vi "Send Menu Selection.vi"(4 "Item Path":string, 5 "EventFilter Reference":T1, 6 "Item Tag":string, 7 "App Item?":bool, 8 "Time":u32, 9 "MenuRef":refnum<k9>, 10 "VI Refnum":refnum<vi>, 11 "Message Enqueuer in":refnum<class "Message Enqueuer.lvclass">) -> (0 "error out":errorcluster, 3 "Filtered EventDataMessage":refnum<class "MenuSelectionMsg.lvclass">)   [LabVIEW 2018, in "MVA Framework.lvlib" / "ActorEvents.lvlib" / "MenuSelectionMsg.lvclass"]
doc: "<License>\nCopyright © 2017 Composed Systems, LLC | All rights reserved\nwww.composed.io\n\nAuthor: Ethan Stern <ethan.stern@composed.io>\n\nThis software is provided \"AS IS\" WITHOUT WARRANTIES, either express or implied, AND IS FOR EDUCATIONAL PURPOSES ONLY.\n</License>"
uses:
  MenuSelectionMsg.lvclass
  EventDataMessage/EventDataMessage.lvclass
  <vilib>/ActorFramework/Message Enqueuer/Message Enqueuer.lvclass
  IEventFilter/IEventFilter.lvclass
  IEventFilter/EventFilter Reference.ctl
panel:
  in  "error in (no error)":errorcluster
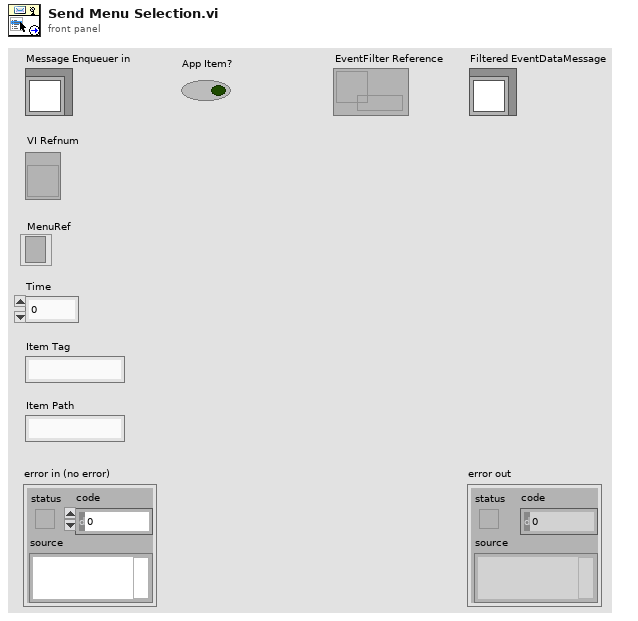
[diagram p1: front panel]
types:
  T1 = typedef "MVA Framework.lvlib/ActorEvents.lvlib/IEventFilter.lvclass/EventFilter Reference.ctl" = refnum<data-value>
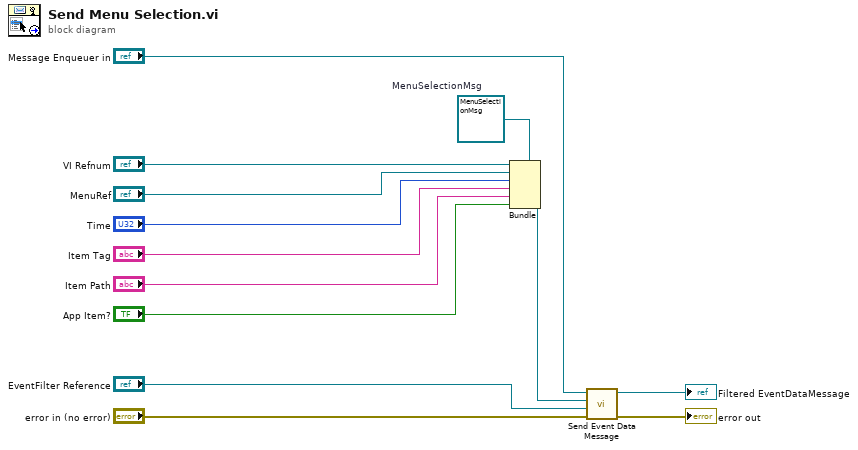
[diagram p0: block diagram]
diagram:
  w13 = refnum<class "MenuSelectionMsg.lvclass"> refnum  # MenuSelectionMsg
  n1 = Bundle(cluster=w13, "VI Refnum", "MenuRef", "Time", "Item Tag", "Item Path", "App Item?") -> (w10:refnum<class "MenuSelectionMsg.lvclass">)
  n2 = call "Send Event Data Message.vi"("error in (no error)"="error in (no error)", "EventFilter Reference"="EventFilter Reference", "EventDataMessage"=w10, "Message Enqueuer in"="Message Enqueuer in") -> ("error out"=→"error out":errorcluster, "Filtered EventDataMessage"=→"Filtered EventDataMessage":refnum<class "MenuSelectionMsg.lvclass">)  [unwired: 6 in]
